vi "Webcam.vi"() -> ()   [LabVIEW 2020]
uses:
  State_Variables.ctl
  States.ctl
  System.Windows.Forms
panel:
  in  "Tab Control":enum32{"Interface", "Debug"}(tab)
  in  "stop":bool
  in  "PictureBox":refnum<k24>(container)
  in  "Default State Variables":T1={"Window Title"="\"Window Title\""}
  out "error out":errorcluster
  out "Current Values":T1
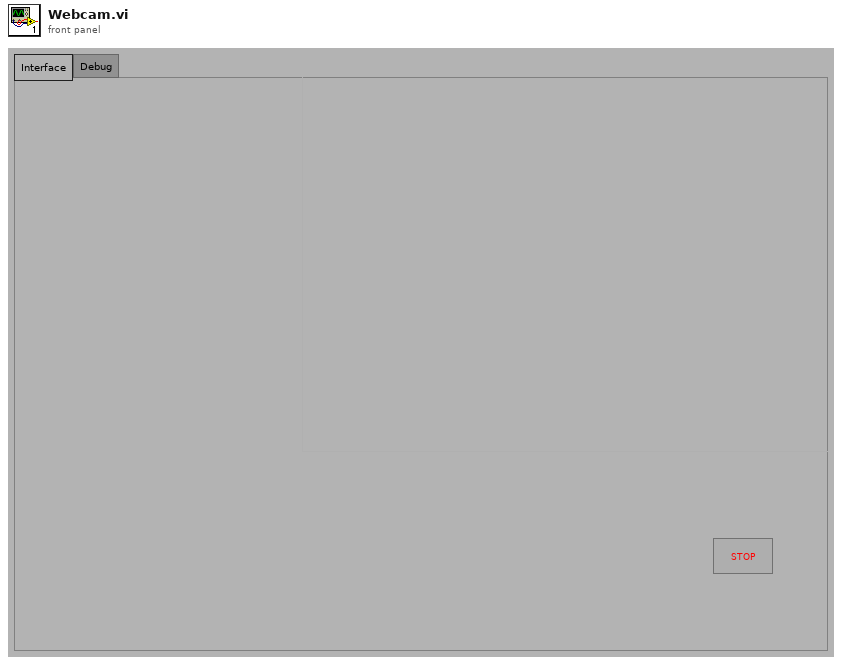
[diagram p1: front panel]
types:
  T1 = typedef "State_Variables.ctl" = cluster{"Window Title":string}
  T2 = typedef "States.ctl" = enum16{"Waiting", "Init", "Cleanup", "Exit", "Init1", "Init2"}
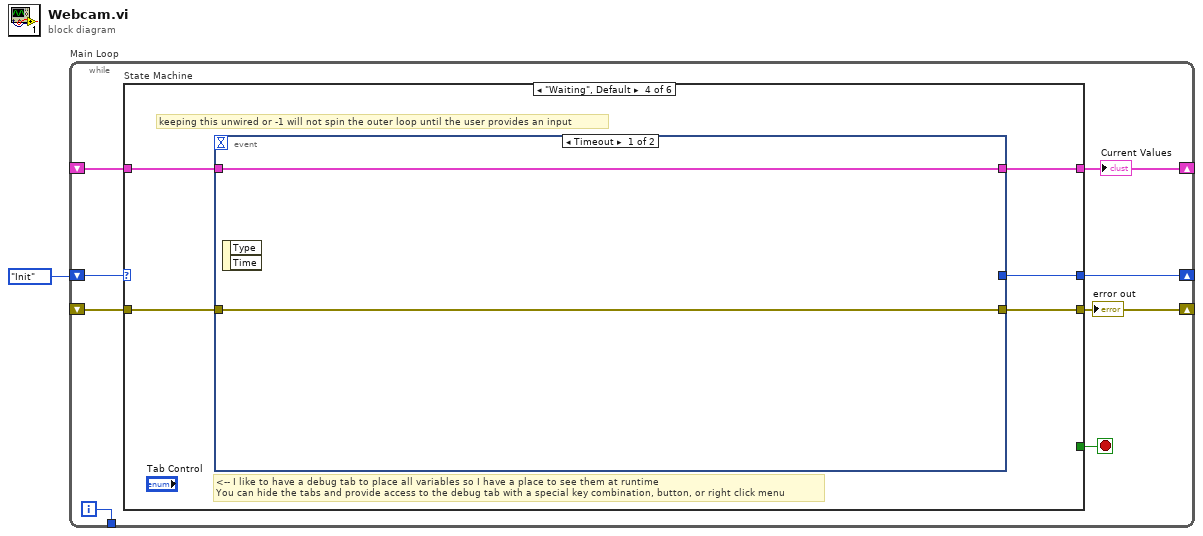
[diagram p0: block diagram]
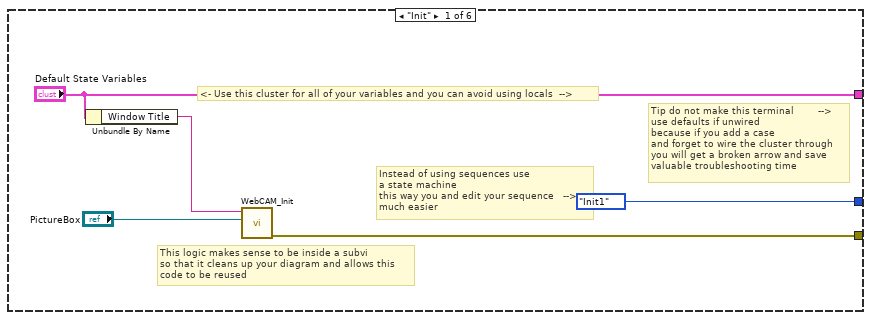
[diagram p2: hidden frame]
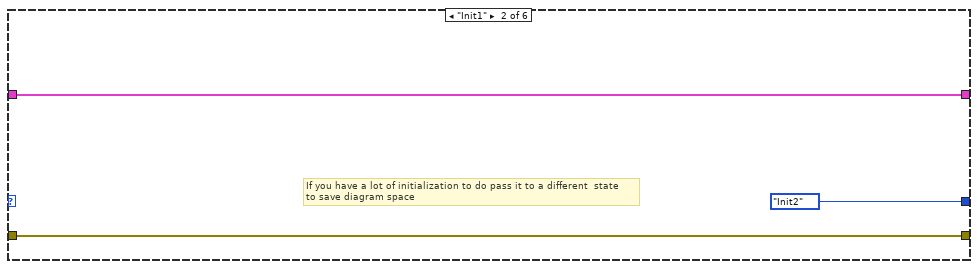
[diagram p3: hidden frame]
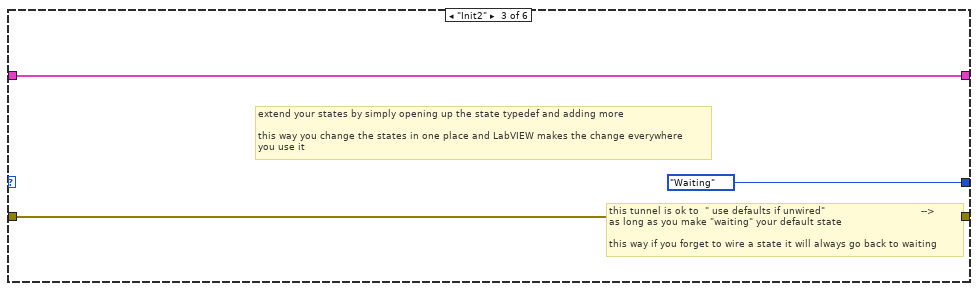
[diagram p4: hidden frame]
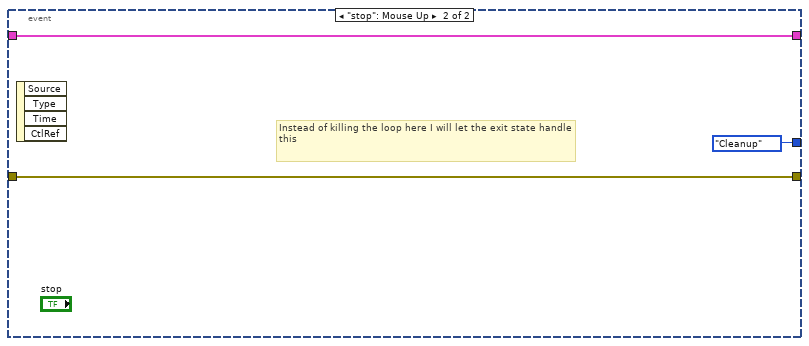
[diagram p5: hidden frame]
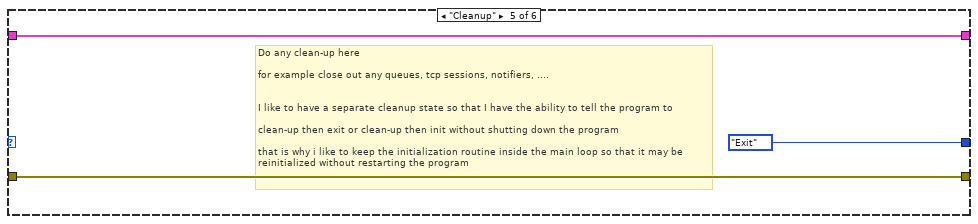
[diagram p6: hidden frame]
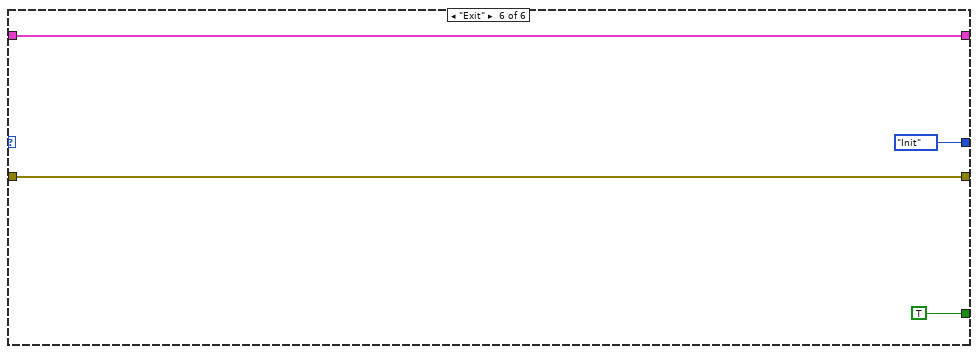
[diagram p7: hidden frame]
diagram:
  n1 = while "Main Loop" {
    shift-right: [w4] -> _
    shift-left: States."Init" ("States") -> [w8]
    tunnel: [w7] -> _
    shift-right: [w5] -> _
    shift-left: _ -> [w6]
    shift-right: [w3] -> _
    shift-left: _ -> [w2]
    i -> [w7]
    stop <- w9 stop-if-true
    n2 = case "State Machine" shown="\"Waiting\", Default" w8 {
      tunnel: [_ _ _ _ _ TRUE] -> w9
      tunnel: w6 -> [_ w17 w20 w25 w33 w37]
      tunnel: [w13 w17 w20 w24 w33 w37] -> w5
      tunnel: [States."Init1" ("States") States."Init2" ("States") States."Waiting" ("States") w21 States."Exit" ("States") States."Init" ("States")] -> w4
      tunnel: ["Default State Variables" w15 w18 w22 w31 w36] -> w3
      tunnel: w2 -> [_ w15 w18 w23 w31 w36]
      frame "Init" {
        # "This logic makes sense to be inside a subvi\nso that it cleans up your diagram and allows this \ncode to be reused"
        # "Instead of using sequences use  \na state machine\nthis way you and edit your sequence   -->\nmuch easier"
        # "Tip do not make this terminal        --> \nuse defaults if unwired\nbecause if you add a case\nand forget to wire the cluster through\nyou will get a broken arrow and save\nvaluable troubleshooting time"
        # "<- Use this cluster for all of your variables and you can avoid using locals  -->"
        n3 = Unbundle By Name("Default State Variables") -> ("Window Title"=w11:string)
        n4 = call "WebCAM_Init.vi"("PictureBox"="PictureBox", "Window Title"=w11) -> ("error out"=w13:errorcluster)  [unwired: 9 in]
      }
      frame "Init1" {
        # "If you have a lot of initialization to do pass it to a different  state\nto save diagram space"
      }
      frame "Init2" {
        # "this tunnel is ok to  \" use defaults if unwired\"                                -->\nas long as you make \"waiting\" your default state\n\nthis way if you forget to wire a state it will always go back to waiting"
        # "extend your states by simply opening up the state typedef and adding more\n\nthis way you change the states in one place and LabVIEW makes the change everywhere\nyou use it"
      }
      frame "Waiting", Default {
        # "<-- I like to have a debug tab to place all variables so I have a place to see them at runtime\nYou can hide the tabs and provide access to the debug tab with a special key combination, button, or right click menu"
        # "keeping this unwired or -1 will not spin the outer loop until the user provides an input"
        n5 = event shown="[0] Timeout" {
          selector: _ -> [_ _]
          dyn-events: _ -> [_ _]
          timeout: _ -> [_ _]
          tunnel: w25 -> [w27 w30]
          tunnel: [w27 w30] -> w24
          tunnel: w23 -> [w26 w29]
          tunnel: [w26 w29] -> w22
          tunnel: [_ w28] -> _
          tunnel: [_ w28] -> w21
          event Timeout {
            n6 = event-data() -> ()  [unwired: 1 in, 2 out]
          }
          event "stop": Mouse Up {
            w28 = States."Cleanup" ("States")
            # "Instead of killing the loop here I will let the exit state handle this"
            n7 = event-data() -> ()  [unwired: 1 in, 4 out]
          }
        }
      }
      frame "Cleanup" {
        # "Do any clean-up here \n\nfor example close out any queues, tcp sessions, notifiers, ....\n\n\nI like to have a separate cleanup state so that I have the ability to tell the program to \n\nclean-up then exit or clean-up then init without shutting down the program\n\nthat is why i like to keep the initialization routine inside the main loop so that it may be \nreinitialized without restarting the program"
      }
      frame "Exit" {
      }
    }
    "error out" <- w5
    "Current Values" <- w3
  }
